vi "Get Version from Git.vi"(8 "error in":errorcluster, 11 "lvlib path":path) -> (0 "error out":errorcluster, 1 "Commit Hash":string, 2 "Version":cluster{i32, i32, i32, i32})   [LabVIEW 2019]
panel:
  in  "index":i32
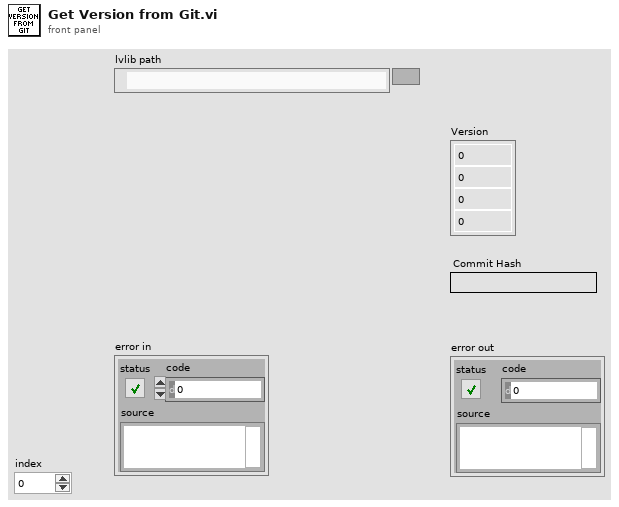
[diagram p1: front panel]
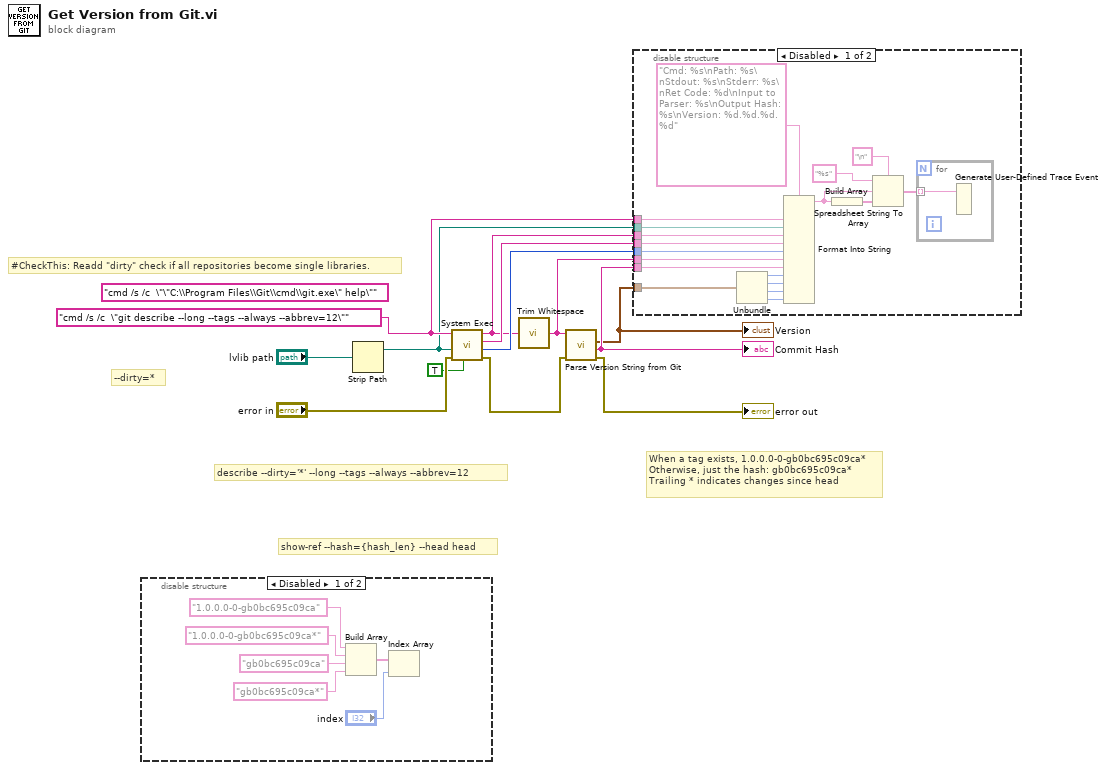
[diagram p0: block diagram]
diagram:
  w8 = "cmd /s /c  \"git describe --long --tags --always --abbrev=12\"" ("command line")
  (unwired) "cmd /s /c  \"\"C:\\Program Files\\Git\\cmd\\git.exe\" help\"" ("command line")
  # "#CheckThis: Readd \"dirty\" check if all repositories become single libraries."
  # "--dirty=*"
  # "show-ref --hash={hash_len} --head head"
  # "When a tag exists, 1.0.0.0-0-gb0bc695c09ca*\nOtherwise, just the hash: gb0bc695c09ca*\nTrailing * indicates changes since head"
  # "describe --dirty='*' --long --tags --always --abbrev=12"
  n1 = disable-structure shown="Disabled" {
    frame Disabled {
      n2 = Build Array("1.0.0.0-0-gb0bc695c09ca", "1.0.0.0-0-gb0bc695c09ca*", "gb0bc695c09ca", "gb0bc695c09ca*") -> (w15:string[])
      n3 = Index Array(array=w15, index="index") -> ()  [unwired: 1 out]
    }
    frame Enabled {
    }
  }
  n4 = Strip Path(path="lvlib path") -> (stripped path=w7:path)  [unwired: 1 out]
  n5 = call <vilib>:"System Exec.vi"("run minimized? (F)"=TRUE, "error in (no error)"="error in", "working directory"=w7, "command line"=w8) -> ("error out"=w10:errorcluster, "return code"=w4:i32, "standard error"=w6:string, "standard output"=w1:string)  [unwired: 4 in]
  n6 = call <vilib>:"Trim Whitespace.vi"("string"=w1) -> ("trimmed string"=w5:string)  [unwired: 1 in]
  n7 = call "Parse Version String from Git.vi"("error in"=w10, "Version String"=w5) -> ("error out"=→"error out":errorcluster, "Commit Hash"=w3:string, "Version"=w2:cluster{i32, i32, i32, i32})  [unwired: 7 in]
  "Version" <- w2
  "Commit Hash" <- w3
  n8 = disable-structure shown="Disabled" {
    disable-tunnel: w8 -> [w36 _]
    disable-tunnel: w7 -> [w35 _]
    disable-tunnel: w6 -> [w34 _]
    disable-tunnel: w5 -> [w33 _]
    disable-tunnel: w4 -> [w32 _]
    disable-tunnel: w3 -> [w31 _]
    disable-tunnel: w2 -> [w30 _]
    disable-tunnel: w1 -> [w20 _]
    frame Disabled {
      n9 = Unbundle(w30) -> (w29:i32, w28:i32, w27:i32, w26:i32)
      n10 = Format Into String(format string="Cmd: %s\nPath: %s\nStdout: %s\nStderr: %s\nRet Code: %d\nInput to Parser: %s\nOutput Hash: %s\nVersion: %d.%d.%d.%d", w36, w35, w20, w34, w32, w33, w31, w29, w28, w27, w26) -> (resulting string=w25:string)  [unwired: 2 in, 1 out]
      n11 = Build Array(w25) -> (w24:string[])
      n12 = Spreadsheet String To Array(delimiter (Tab)="\n", format string="%s", spreadsheet string=w25, array type (2D Dbl)=w24) -> (array=w21:string[])
      n13 = for {
        tunnel: w21 -> [w38] mode=indexing
        n14 = Generate User-Defined Trace Event(2:w38) -> ()  [unwired: 1 in]
      }
    }
    frame Enabled {
    }
  }
